vi "laserNKT_main.vi"() -> ()   [LabVIEW 2011]
panel:
  out "OutParameters":T1 {"Crc16" format="%.0x"; "(hi.lo)" format="%x"; "Register" format="%x"}
  in  "InParameters":T2={"Destination"=2, "Source"=162, "Register"=16, "Array"=[], "WriteNotRead"=FALSE, "ReadWithPreample"=FALSE, "Ring"=0, "String"="", "Long"=0} {"Ring" items=["ByteArray", "IntegerArray", "String", "Long", "Direct string sent"]; "Register" format="%x"}
  in  "PortParameters":T3={"OpenPort"=FALSE, "ClosePort"=FALSE, "Baudrate"=115200, "Wait"=50, "ReadWrite"=FALSE}
  out "appended array":bool[](array[boolean])
  in  "100percent":bool
  in  "75percent":bool
  in  "50percent":bool
  in  "25percent":bool
  in  "power 0":bool
  in  "Set Power (%)":i32 max=2350
  out "Power":i32
  out "Current Power":u8(slide) scale=0.0..100.0
  out "max Q":i32
  out "error out":errorcluster
  in  "Laser COM PORT":refnum<visa-resource-name>="COM14"
  out "MachineState":string="init"
  in  "Emission":bool
  in  "stop":bool
  # "SET POWER"
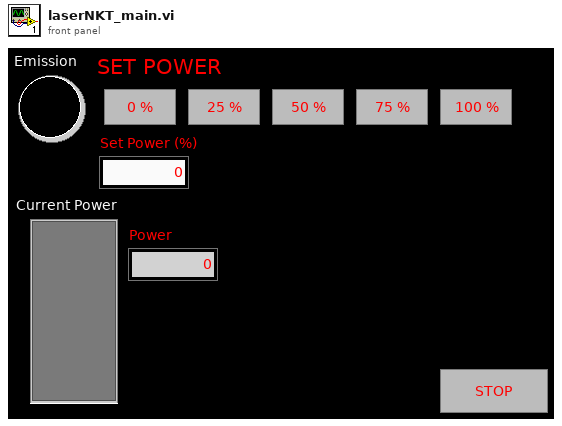
[diagram p1: front panel]
types:
  T1 = cluster{"Source":u8, "TelegramType":u8, "Register":u8, "Destination":u8, "TelegramReceived":bool, "CRC error":bool, "PayloadByteArray":u8[], "(hi.lo)":u16, "Crc16":u16, "Long":i32, "PayloadIntArray":u16[], "String":string}
  T2 = cluster{"Destination":u8, "Source":u8, "Register":u8, "Array":i16[], "WriteNotRead":bool, "ReadWithPreample":bool, "Ring":u16, "String":string, "Long":i32}
  T3 = cluster{"OpenPort":bool, "ClosePort":bool, "Baudrate":i32, "Wait":u16, "ReadWrite":bool}
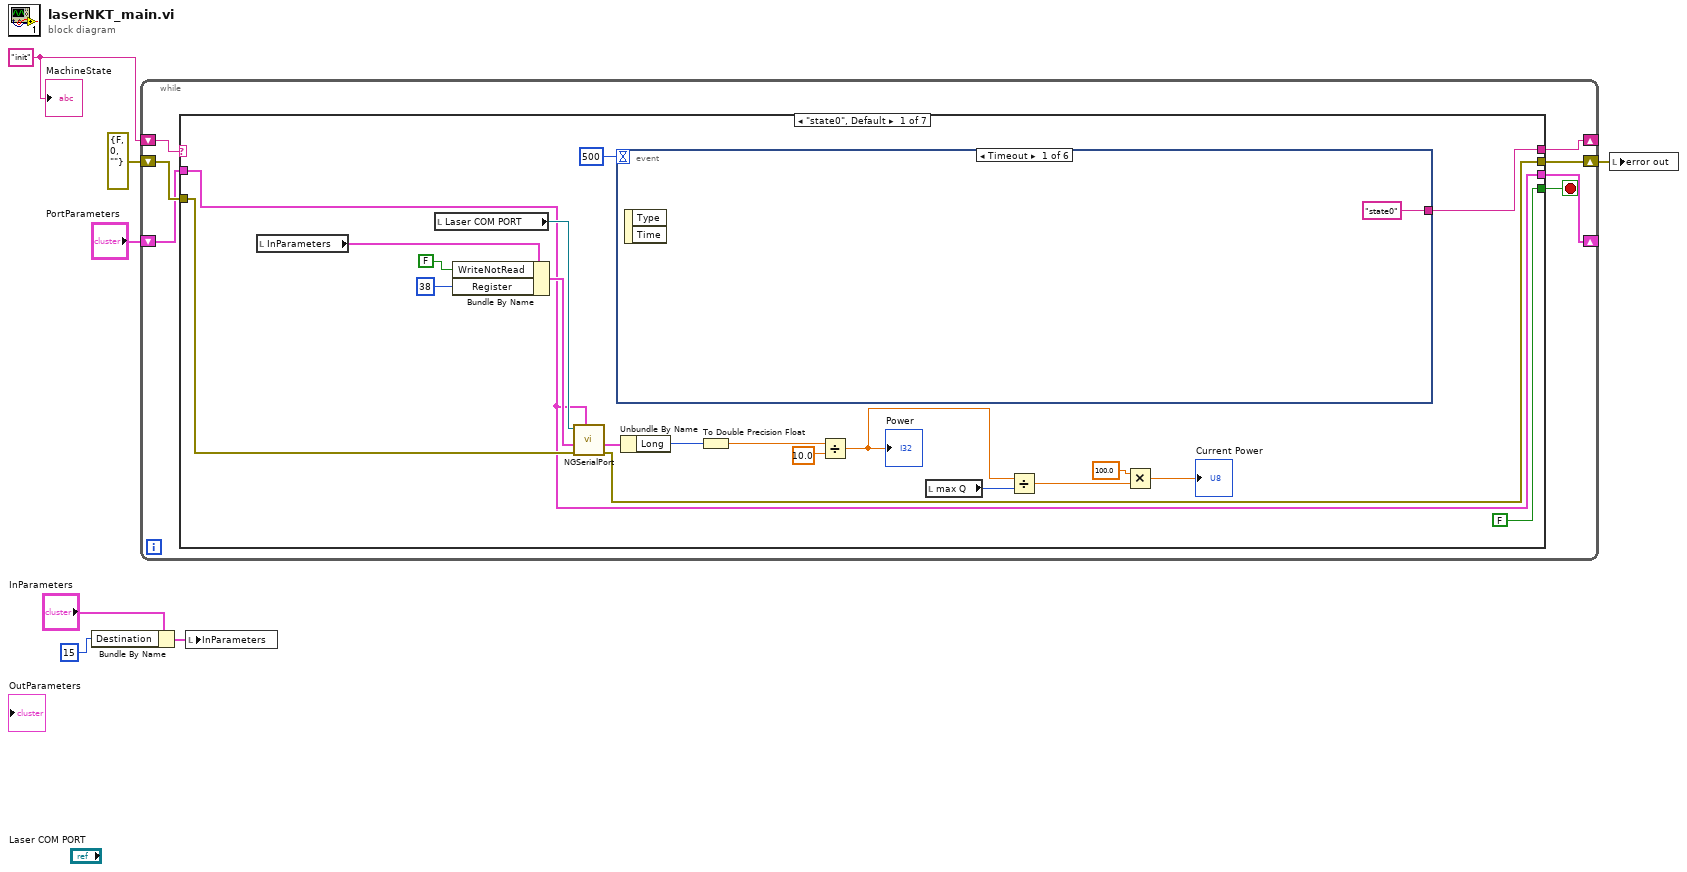
[diagram p0: block diagram]
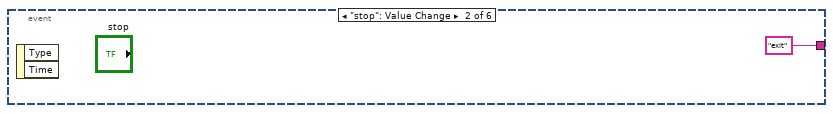
[diagram p2: hidden frame]
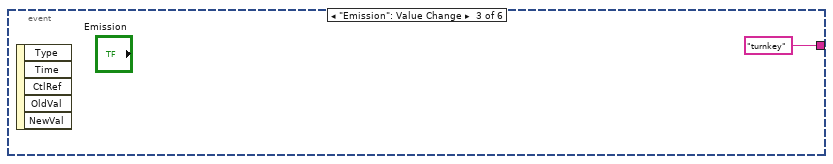
[diagram p3: hidden frame]
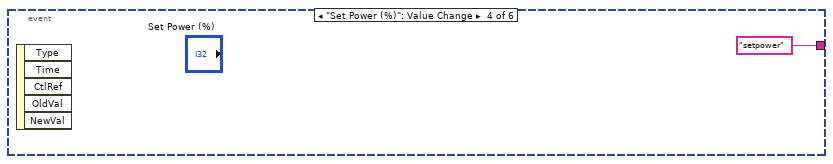
[diagram p4: hidden frame]
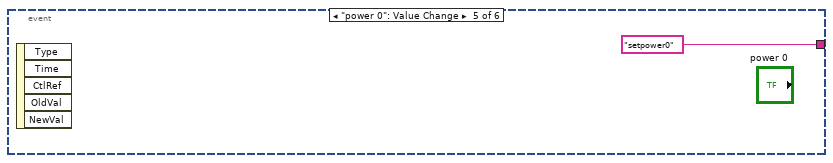
[diagram p5: hidden frame]
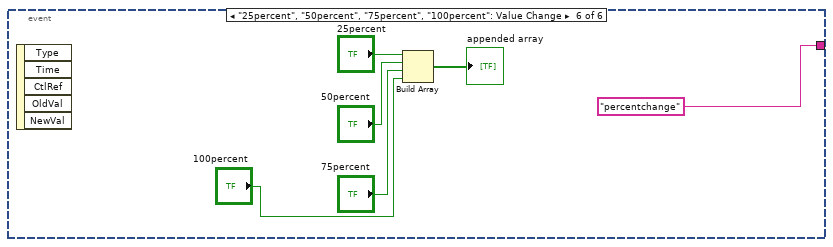
[diagram p6: hidden frame]
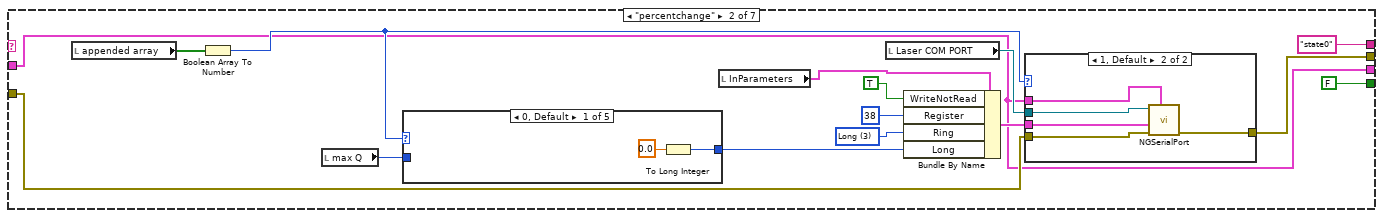
[diagram p7: hidden frame]
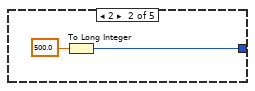
[diagram p9: hidden frame]
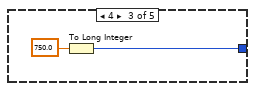
[diagram p10: hidden frame]
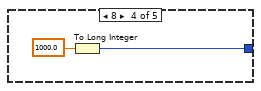
[diagram p11: hidden frame]
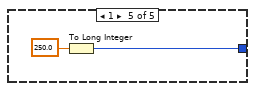
[diagram p12: hidden frame]
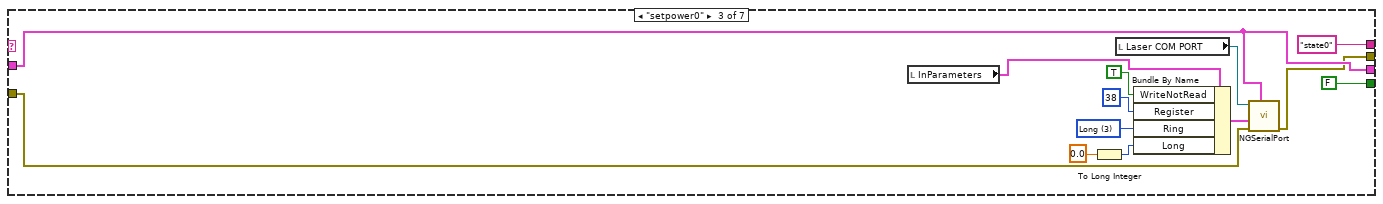
[diagram p13: hidden frame]
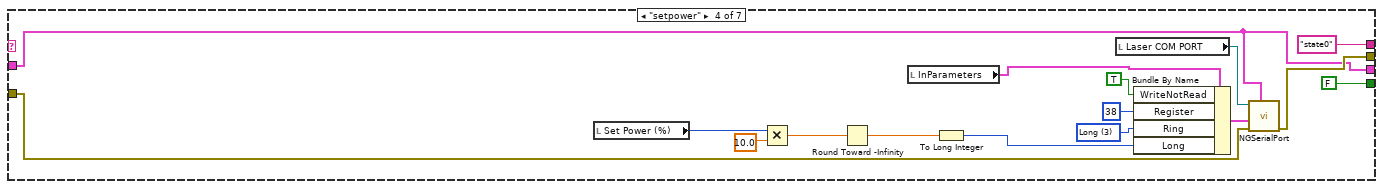
[diagram p14: hidden frame]
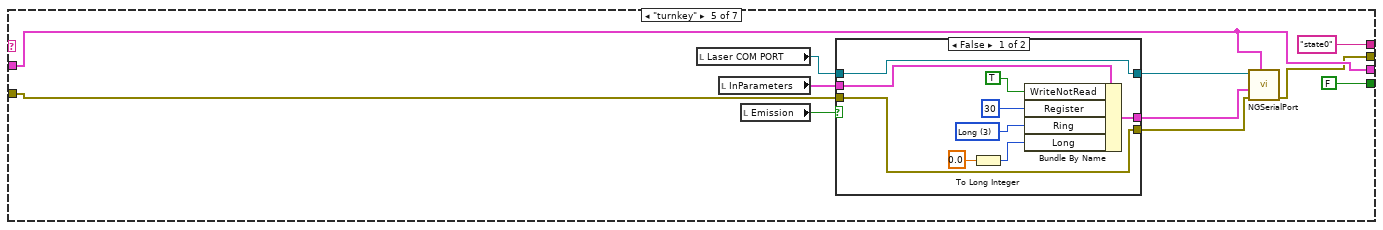
[diagram p15: hidden frame]
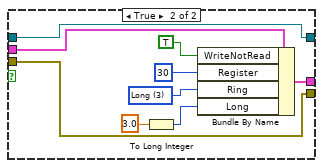
[diagram p16: hidden frame]
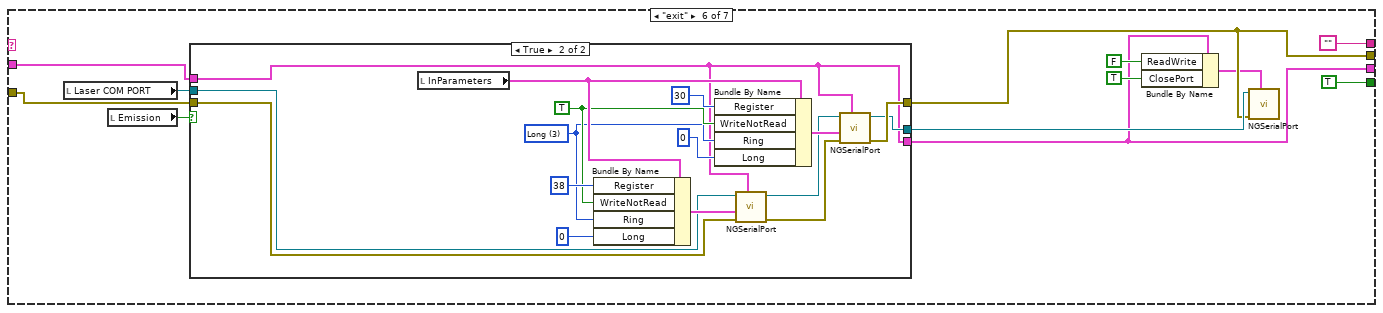
[diagram p17: hidden frame]
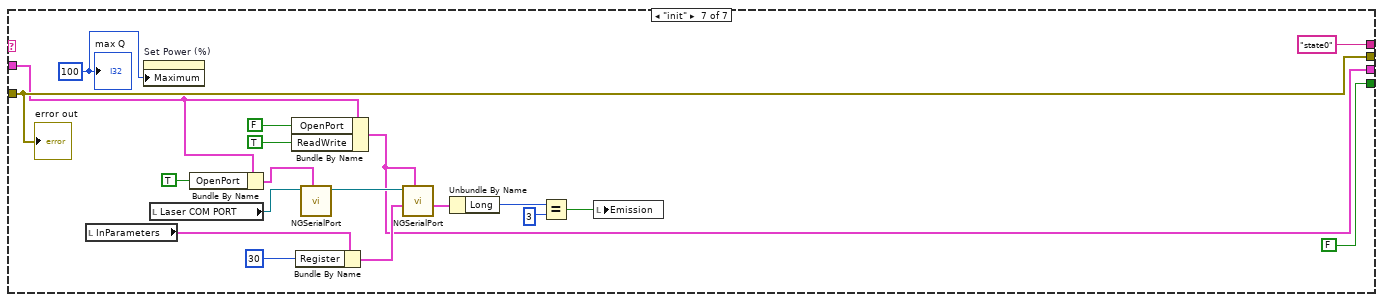
[diagram p19: hidden frame]
diagram:
  w7 = "init"
  n1 = Bundle By Name(cluster="InParameters", "Destination"=u8 15) -> (w3:T2)
  n2 = while {
    shift-right: [w13] -> _
    shift-left: w7 -> [w14]
    shift-right: [w11] -> w6
    shift-left: errorcluster {"status"=FALSE, "code"=0, "source"=""} ("error out") -> [w10]
    shift-right: [w8] -> _
    shift-left: "PortParameters" -> [w9]
    stop <- w12 stop-if-true
    n3 = case shown="\"state0\", Default" w14 {
      tunnel: [w34 "state0" "state0" "state0" "state0" "" "state0"] -> w13
      tunnel: [FALSE FALSE FALSE FALSE FALSE TRUE FALSE] -> w12
      tunnel: [w16 w47 w77 w96 w110 w138 w181] -> w11
      tunnel: w10 -> [w22 w48 w78 w97 w113 w142 w181]
      tunnel: w9 -> [w15 w46 w79 w90 w111 w137 w167]
      tunnel: [w15 w46 w79 w90 w111 w135 w166] -> w8
      frame "state0", Default {
        n4 = local read "InParameters"() -> (w26:T2)
        n5 = local read "Laser COM PORT"() -> (w27:refnum<visa-resource-name>)
        n6 = Bundle By Name(cluster=w26, "WriteNotRead"=FALSE, "Register"=u8 38) -> (w23:T2)
        n7 = call "NGSerialPort.vi"("PortParameters"=w15, "error in"=w22, "InParameters"=w23, "VISA in"=w27) -> ("error out"=w16:errorcluster, "OutParameters"=w21:T1)  [unwired: 5 in, 1 out]
        n8 = event shown="[0] Timeout" {
          selector: _ -> [_ _ _ _ _ _]
          dyn-events: _ -> [_ _ _ _ _ _]
          timeout: 500 -> [_ _ _ _ _ _]
          tunnel: ["state0" "exit" "turnkey" "setpower" "setpower0" "percentchange"] -> w34
          event Timeout {
            n9 = event-data() -> ()  [unwired: 1 in, 2 out]
          }
          event "stop": Value Change {
            n10 = event-data() -> ()  [unwired: 1 in, 2 out]
          }
          event "Emission": Value Change {
            n11 = event-data() -> ()  [unwired: 1 in, 5 out]
          }
          event "Set Power (%)": Value Change {
            n12 = event-data() -> ()  [unwired: 1 in, 5 out]
          }
          event "power 0": Value Change {
            n13 = event-data() -> ()  [unwired: 1 in, 5 out]
          }
          event "25percent", "50percent", "75percent", "100percent": Value Change {
            n14 = event-data() -> ()  [unwired: 1 in, 5 out]
            n15 = Build Array("25percent", "50percent", "75percent", "100percent") -> (→"appended array":bool[])
          }
        }
        n16 = Unbundle By Name(w21) -> ("Long"=w20:i32)
        n17 = To Double Precision Float(number=w20) -> (double precision float=w19:dbl)
        n18 = Divide(x=w19, y=10.0) -> (x/y=w17:dbl)
        "Power" <- w17
        n19 = local read "max Q"() -> (w33:i32)
        n20 = Divide(x=w17, y=w33) -> (x/y=w32:dbl)
        n21 = Multiply(x=100.0, y=w32) -> (x*y=→"Current Power":dbl)
      }
      frame "percentchange" {
        w52 = u16 3 items=["ByteArray", "IntegerArray", "String", "Long", "Direct string sent"] ("Ring")
        n22 = local read "appended array"() -> (w59:bool[])
        n23 = Boolean Array To Number(Boolean array=w59) -> (number=w51:u32)
        n24 = local read "max Q"() -> (w58:i32)
        n25 = case shown="0, Default" w51 {
          tunnel: w58 -> [_ _ _ _ _]
          tunnel: [w67 w69 w71 w73 w75] -> w53
          frame 0, Default {
            n26 = To Long Integer(number=0.0) -> (32bit integer=w67:i32)
          }
          frame 2 {
            n27 = To Long Integer(number=500.0) -> (32bit integer=w69:i32)
          }
          frame 4 {
            n28 = To Long Integer(number=750.0) -> (32bit integer=w71:i32)
          }
          frame 8 {
            n29 = To Long Integer(number=1000.0) -> (32bit integer=w73:i32)
          }
          frame 1 {
            n30 = To Long Integer(number=250.0) -> (32bit integer=w75:i32)
          }
        }
        n31 = local read "InParameters"() -> (w54:T2)
        n32 = local read "Laser COM PORT"() -> (w49:refnum<visa-resource-name>)
        n33 = Bundle By Name(cluster=w54, "WriteNotRead"=TRUE, "Register"=u8 38, "Ring"=w52, "Long"=w53) -> (w50:T2)
        n34 = case shown="1, Default" w51 {
          tunnel: w50 -> [_ w66]
          tunnel: w49 -> [_ w65]
          tunnel: w48 -> [w61 w64]
          tunnel: [w61 w63] -> w47
          tunnel: w46 -> [_ w62]
          frame 0 {
          }
          frame 1, Default {
            n35 = call "NGSerialPort.vi"("PortParameters"=w62, "error in"=w64, "InParameters"=w66, "VISA in"=w65) -> ("error out"=w63:errorcluster)  [unwired: 5 in, 2 out]
          }
        }
      }
      frame "setpower0" {
        w85 = u16 3 items=["ByteArray", "IntegerArray", "String", "Long", "Direct string sent"] ("Ring")
        n36 = local read "InParameters"() -> (w80:T2)
        n37 = To Long Integer(number=0.0) -> (32bit integer=w82:i32)
        n38 = local read "Laser COM PORT"() -> (w81:refnum<visa-resource-name>)
        n39 = Bundle By Name(cluster=w80, "WriteNotRead"=TRUE, "Register"=u8 38, "Ring"=w85, "Long"=w82) -> (w83:T2)
        n40 = call "NGSerialPort.vi"("PortParameters"=w79, "error in"=w78, "InParameters"=w83, "VISA in"=w81) -> ("error out"=w77:errorcluster)  [unwired: 5 in, 2 out]
      }
      frame "setpower" {
        w101 = u16 3 items=["ByteArray", "IntegerArray", "String", "Long", "Direct string sent"] ("Ring")
        n41 = local read "Set Power (%)"() -> (w95:i32)
        n42 = Multiply(x=w95, y=10.0) -> (x*y=w93:dbl)
        n43 = Round Toward -Infinity(1:w93) -> (0:w92:dbl)
        n44 = local read "InParameters"() -> (w91:T2)
        n45 = To Long Integer(number=w92) -> (32bit integer=w99:i32)
        n46 = local read "Laser COM PORT"() -> (w98:refnum<visa-resource-name>)
        n47 = Bundle By Name(cluster=w91, "WriteNotRead"=TRUE, "Register"=u8 38, "Ring"=w101, "Long"=w99) -> (w100:T2)
        n48 = call "NGSerialPort.vi"("PortParameters"=w90, "error in"=w97, "InParameters"=w100, "VISA in"=w98) -> ("error out"=w96:errorcluster)  [unwired: 5 in, 2 out]
      }
      frame "turnkey" {
        n49 = local read "Laser COM PORT"() -> (w114:refnum<visa-resource-name>)
        n50 = local read "InParameters"() -> (w109:T2)
        n51 = local read "Emission"() -> (w115:bool)
        n52 = case shown="False" w115 {
          tunnel: w114 -> [w117 w134]
          tunnel: [w117 w134] -> w106
          tunnel: w113 -> [w125 w133]
          tunnel: [w125 w133] -> w107
          tunnel: w109 -> [w119 w127]
          tunnel: [w118 w126] -> w108
          frame False {
            w122 = u16 3 items=["ByteArray", "IntegerArray", "String", "Long", "Direct string sent"] ("Ring")
            n53 = To Long Integer(number=0.0) -> (32bit integer=w120:i32)
            n54 = Bundle By Name(cluster=w119, "WriteNotRead"=TRUE, "Register"=u8 30, "Ring"=w122, "Long"=w120) -> (w118:T2)
          }
          frame True {
            w130 = u16 3 items=["ByteArray", "IntegerArray", "String", "Long", "Direct string sent"] ("Ring")
            n55 = To Long Integer(number=3.0) -> (32bit integer=w128:i32)
            n56 = Bundle By Name(cluster=w127, "WriteNotRead"=TRUE, "Register"=u8 30, "Ring"=w130, "Long"=w128) -> (w126:T2)
          }
        }
        n57 = call "NGSerialPort.vi"("PortParameters"=w111, "error in"=w107, "InParameters"=w108, "VISA in"=w106) -> ("error out"=w110:errorcluster)  [unwired: 5 in, 2 out]
      }
      frame "exit" {
        n58 = local read "Laser COM PORT"() -> (w144:refnum<visa-resource-name>)
        n59 = local read "Emission"() -> (w143:bool)
        n60 = case shown="True" w143 {
          tunnel: w144 -> [w149 w162]
          tunnel: w142 -> [w148 w154]
          tunnel: [w148 w153] -> w138
          tunnel: [w149 w152] -> w139
          tunnel: w137 -> [w147 w150]
          tunnel: [w147 w150] -> w135
          frame False {
          }
          frame True {
            w151 = u16 3 items=["ByteArray", "IntegerArray", "String", "Long", "Direct string sent"] ("Ring")
            w160 = TRUE ("WriteNotRead")
            n61 = local read "InParameters"() -> (w161:T2)
            n62 = Bundle By Name(cluster=w161, "Register"=u8 38, "WriteNotRead"=w160, "Ring"=w151, "Long"=0) -> (w163:T2)
            n63 = Bundle By Name(cluster=w161, "Register"=u8 30, "WriteNotRead"=w160, "Ring"=w151, "Long"=0) -> (w157:T2)
            n64 = call "NGSerialPort.vi"("PortParameters"=w150, "error in"=w154, "InParameters"=w163, "VISA in"=w162) -> ("error out"=w155:errorcluster, "VISA out"=w156:refnum<visa-resource-name>)  [unwired: 5 in, 1 out]
            n65 = call "NGSerialPort.vi"("PortParameters"=w150, "error in"=w155, "InParameters"=w157, "VISA in"=w156) -> ("error out"=w153:errorcluster, "VISA out"=w152:refnum<visa-resource-name>)  [unwired: 5 in, 1 out]
          }
        }
        n66 = Bundle By Name(cluster=w135, "ReadWrite"=FALSE, "ClosePort"=TRUE) -> (w136:T3)
        n67 = call "NGSerialPort.vi"("PortParameters"=w136, "error in"=w138, "VISA in"=w139) -> ()  [unwired: 6 in, 3 out]
      }
      frame "init" {
        w183 = 100 ("max Q")
        n68 = local read "InParameters"() -> (w174:T2)
        n69 = property on="Set Power (%)" class="DigNum (strict)"("Maximum"=w183) -> ()  [unwired: 2 in, 2 out]
        n70 = local read "Laser COM PORT"() -> (w180:refnum<visa-resource-name>)
        n71 = Bundle By Name(cluster=w167, "OpenPort"=TRUE) -> (w178:T3)
        n72 = Bundle By Name(cluster=w167, "OpenPort"=FALSE, "ReadWrite"=TRUE) -> (w166:T3)
        n73 = Bundle By Name(cluster=w174, "Register"=u8 30) -> (w172:T2)
        n74 = call "NGSerialPort.vi"("PortParameters"=w178, "VISA in"=w180) -> ("VISA out"=w175:refnum<visa-resource-name>)  [unwired: 7 in, 2 out]
        n75 = call "NGSerialPort.vi"("PortParameters"=w166, "InParameters"=w172, "VISA in"=w175) -> ("OutParameters"=w171:T1)  [unwired: 6 in, 2 out]
        n76 = Unbundle By Name(w171) -> ("Long"=w170:i32)
        n77 = Equal?(x=w170, y=3) -> (x = y?=w168:bool)
        n78 = local write "Emission"(w168) -> ()
        "error out" <- w181
        "max Q" <- w183
      }
    }
  }
  n79 = local write "InParameters"(w3) -> ()
  n80 = local write "error out"(w6) -> ()
  "MachineState" <- w7
